vi "DAQ_task_START.vi"(0 "error in":errorcluster) -> (2 "error out":errorcluster)   [LabVIEW 2015]
uses:
  GLOBAL/Global_DAQ.vi
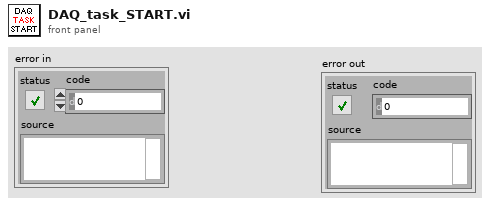
[diagram p1: front panel]
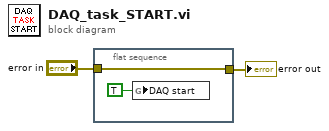
[diagram p0: block diagram]
diagram:
  n1 = flat-sequence {
    tunnel: "error in" -> [w3]
    tunnel: [w3] -> w2
    frame #0 {
      n2 = global write "Global_DAQ.vi" "DAQ start"(TRUE ("Start ANDOR")) -> ()
    }
  }
  "error out" <- w2
